vi "DataToColors.vi"(11 "Label":i32) -> (3 "Color":u32(colorbox))   [LabVIEW 2020]
doc: "Assign a color to a label"
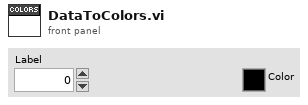
[diagram p1: front panel]
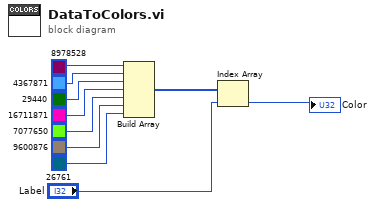
[diagram p0: block diagram]
diagram:
  n1 = Build Array(u32 8978528 ("Color Box"), u32 4367871 ("Color Box"), u32 29440 ("Color Box"), u32 16711871 ("Color Box"), u32 7077650 ("Color Box"), u32 9600876 ("Color Box"), u32 26761 ("Color Box")) -> (w9:u32[])
  n2 = Index Array(array=w9, index="Label") -> (element=→"Color":u32)
